vi "Retrieve SubComponent Data.vi"(5 "Component ID":u8, 7 "FPGA Interface":refnum<class "FPGA Interface.lvclass">, 8 "error in (no error)":errorcluster, 11 "Bus Monitor in":refnum<class "Bus Monitor.lvclass">) -> (0 "error out":errorcluster, 3 "Bus Monitor out":refnum<class "Bus Monitor.lvclass">)   [LabVIEW 2020, in "BCI-1553 API.lvlib" / "Bus Monitor.lvclass"]
doc: "Retrieves the most recent transacted data values present for each parameter in each filter."
uses:
  Bus Monitor.lvclass
  Dependencies/FPGA Interface/FPGA Interface.lvclass
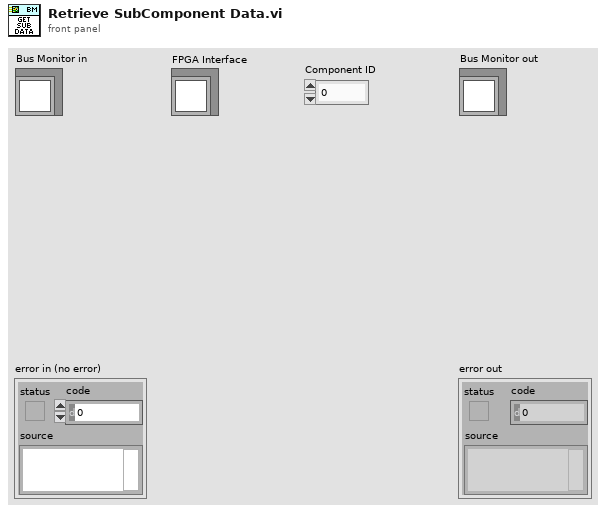
[diagram p1: front panel]
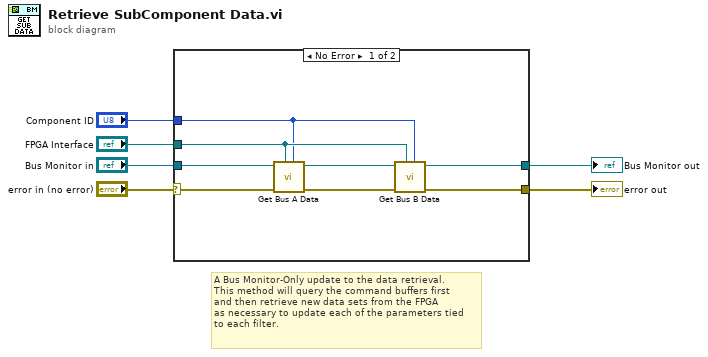
[diagram p0: block diagram]
diagram:
  # "A Bus Monitor-Only update to the data retrieval.\nThis method will query the command buffers first\nand then retrieve new data sets from the FPGA\nas necessary to update each of the parameters tied\nto each filter."
  n1 = case shown="No Error" "error in (no error)" {
    selector: "error in (no error)" -> [w10 w16]
    tunnel: [w9 w16] -> w5
    tunnel: [w12 w15] -> w4
    tunnel: "Bus Monitor in" -> [w13 w15]
    tunnel: "FPGA Interface" -> [w8 _]
    tunnel: "Component ID" -> [w7 _]
    frame No Error {
      n2 = call "Get Bus A Data.vi"("Component ID"=w7, "FPGA Interface"=w8, "error in (no error)"=w10, "Bus Monitor in"=w13) -> ("error out"=w11:errorcluster, "Bus Monitor out"=w14:refnum<class "Bus Monitor.lvclass">)  [unwired: 6 in]
      n3 = call "Get Bus B Data.vi"("Component ID"=w7, "FPGA Interface"=w8, "error in (no error)"=w11, "Bus Monitor in"=w14) -> ("error out"=w9:errorcluster, "Bus Monitor out"=w12:refnum<class "Bus Monitor.lvclass">)  [unwired: 6 in]
    }
    frame Error {
    }
  }
  "error out" <- w5
  "Bus Monitor out" <- w4
